vi "Autonomous Independent.vi"() -> ()   [LabVIEW 2016]
doc: "This VI is called when autonomous begins, and will automatically be terminated when autonomous ends. You can carry out timed or sensor driven robot movement independently without needing to return to the caller."
uses:
  <vilib>/Rock Robotics/WPI/Utilities/WPI_GetSetVariantRefNum.vi
  <vilib>/Rock Robotics/Network Tables/NT Read String.vi
  <vilib>/Rock Robotics/WPI/RobotDrive/WPI_RobotDriveArcadeDrive_Standard(NoSaturation).vi
  <vilib>/Rock Robotics/Network Tables/NT Write Numeric Array.vi
  <vilib>/Rock Robotics/WPI/Solenoid/WPI_SolenoidValue.ctl
  <vilib>/Rock Robotics/WPI/Solenoid/WPI_SolenoidSetEnum.vi
panel:
  in  "stop":bool
  in  "Left":dbl=0.5 step=0.1 format="%#_13g"
  in  "Right":dbl=0.45 step=0.1 format="%#_13g"
  # "Be sure to right-click and choose Data Operations>>Make Current Value default if you want to save the array values with the VI"
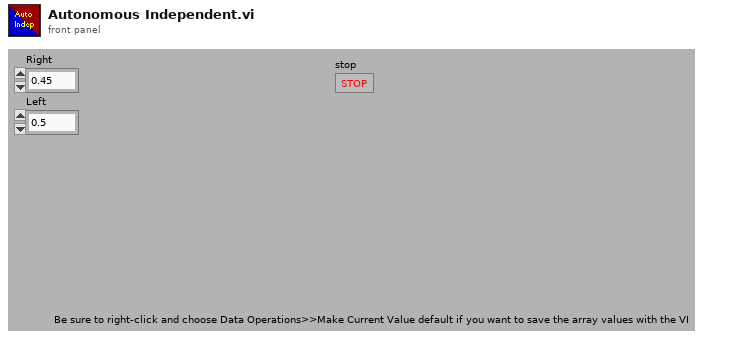
[diagram p1: front panel]
types:
  T1 = typedef "WPI_JoystickDevRef.ctl" = cluster{"Device":T2}
  T2 = typedef "WPI_JoystickDeviceEnum.ctl" = enum16{"USB 0", "USB 1", "USB 2", "USB 3", "USB 4", "USB 5"}
  T3 = typedef "WPI_SolenoidValue.ctl" = enum16{"Off", "On", "Forward", "Reverse"}
  T4 = typedef "WPI_SolenoidDevRef.ctl" = cluster{"DevStatus":errorcluster, "Pneumatics Control Module":u8, "Forward Solenoid Channel":T5, "Reverse Solenoid Channel":T5}
  T5 = typedef "WPI_SolenoidChannel.ctl" = enum8{"Solenoid 0", "Solenoid 1", "Solenoid 2", "Solenoid 3", "Solenoid 4", "Solenoid 5", "Solenoid 6", "Solenoid 7", "Invalid"}
  T6 = typedef "WPI_RobotDriveDevRef.ctl" = cluster{"DevStatus":errorcluster, "Motors[]":T7[], "Square Inputs":bool, "Max Output":dbl}
  T7 = typedef "WPI_MotorControlDeviceRef.ctl" = cluster{"DeviceStatus":errorcluster, "Type":T8, "PWM":cluster{"PWM Channel":T9, "DeadBand":T10}, "CAN":cluster{"Device Number":u8, "SetOutput VI Ref":variant, "GetOutput VI Ref":variant, "Enable VI Ref":variant, "Disable VI Ref":variant, "Data":variant}, "Invert":bool}
  T8 = typedef "WPI_MotorControlType.ctl" = enum16{"PWM", "CAN"}
  T9 = typedef "FPGA_DIOPWMChannel.ctl" = enum8{"PWM 0", "PWM 1", "PWM 2", "PWM 3", "PWM 4", "PWM 5", "PWM 6", "PWM 7", "PWM 8", "PWM 9", "PWM MXP 0", "PWM MXP 1", "PWM MXP 2", "PWM MXP 3", "PWM MXP 4", "PWM MXP 5", "PWM MXP 6", "PWM MXP 7", "PWM MXP 8", "PWM MXP 9", "Invalid"}
  T10 = typedef "WPI_PWMDeadband.ctl" = cluster{"Name":string, "maxPositivePwm":i32, "minPositivePwm":i32, "centerPwm":i32, "maxNegativePwm":i32, "minNegativePwm":i32, "angularRange":u16}
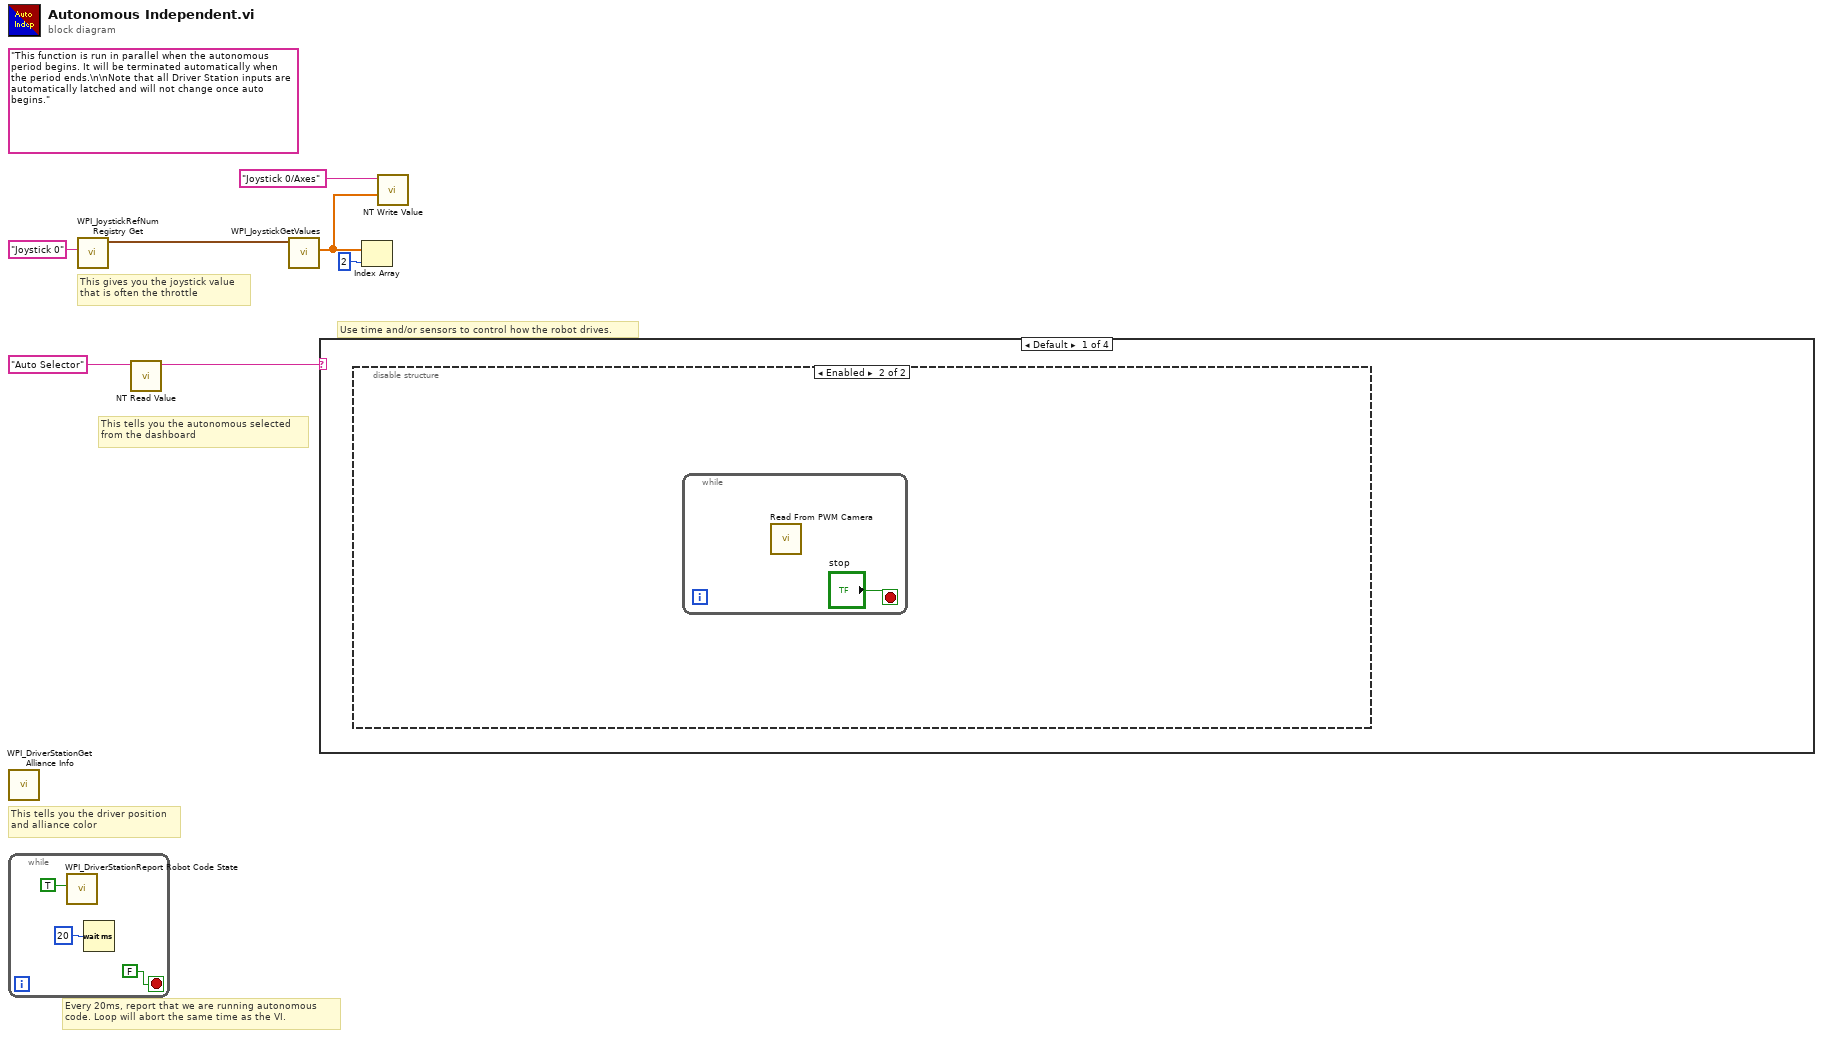
[diagram p0: block diagram]
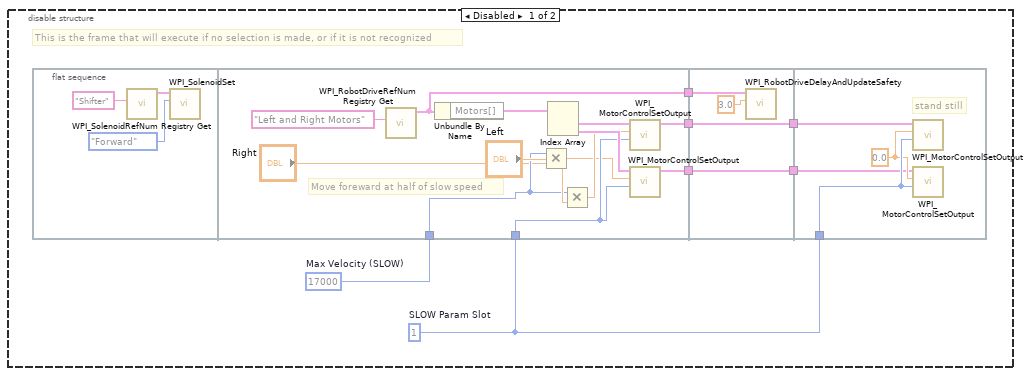
[diagram p2: hidden frame]
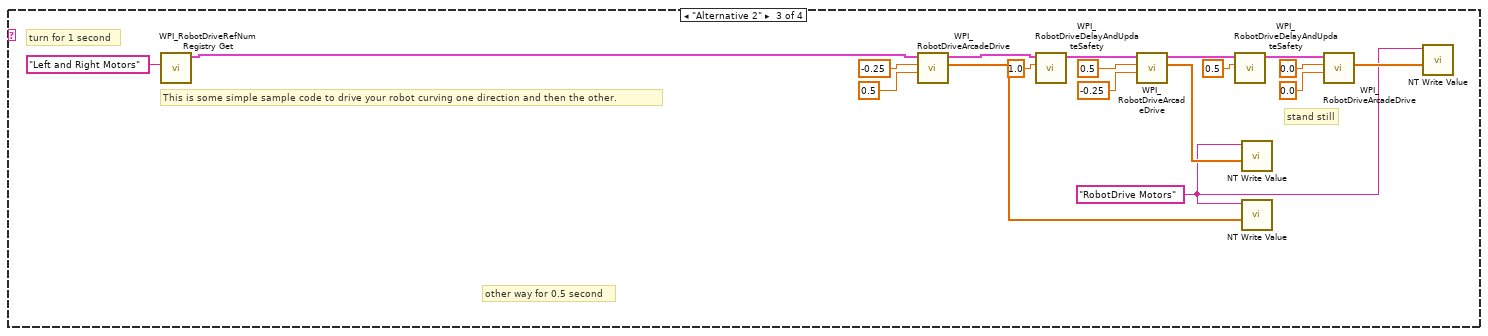
[diagram p4: hidden frame]
diagram:
  (unwired) "This function is run in parallel when the autonomous period begins. It will be terminated automatically when the period ends.\n\nNote that all Driver Station inputs are automatically latched and will not change once auto begins."
  # "This tells you the autonomous selected\nfrom the dashboard"
  # "Every 20ms, report that we are running autonomous\ncode. Loop will abort the same time as the VI."
  # "This gives you the joystick value\nthat is often the throttle"
  # "Use time and/or sensors to control how the robot drives."
  # "This tells you the driver position\nand alliance color"
  n1 = call <vilib>:"WPI_DriverStationGet Alliance Info.vi"() -> ()  [unwired: 12 out]
  n2 = while {
    stop <- FALSE stop-if-true
    n3 = call <vilib>:"WPI_DriverStationReport Robot Code State.vi"("Autonomous"=TRUE) -> ()  [unwired: 10 in, 1 out]
    n4 = Wait (ms)(milliseconds to wait=u32 20) -> ()  [unwired: 1 out]
  }
  n5 = call <vilib>:"WPI_JoystickRefNum Registry Get.vi"("refnum name"="Joystick 0") -> ("JoystickDevRef"=w6:T1)  [unwired: 1 in, 9 out]
  n6 = call-poly <vilib>:"NT Read Value.vi"("Name"="Auto Selector") -> ("String"=w3:string)  [unwired: 9 in, 1 out]
  n7 = call <vilib>:"WPI_JoystickGetValues.vi"("JoystickDevRef"=w6) -> ("Axes"=w2:dbl[])  [unwired: 6 in, 4 out]
  n8 = case shown="Default" w3 {
    frame Default {
      n9 = disable-structure shown="Enabled" {
        frame Disabled {
          w12 = 17000  # Max Velocity (SLOW)
          w11 = 1  # SLOW Param Slot
          # "This is the frame that will execute if no selection is made, or if it is not recognized"
          n10 = flat-sequence {
            tunnel: [w30] -> w17
            tunnel: w11 -> [w27]
            tunnel: w12 -> [w23]
            tunnel: [w25] -> w16
            tunnel: [w24] -> w15
            tunnel: w17 -> [w36]
            tunnel: w16 -> [w35]
            tunnel: [w35] -> w14
            tunnel: w15 -> [w34]
            tunnel: [w34] -> w13
            tunnel: w11 -> [w41]
            tunnel: w14 -> [w39]
            tunnel: w13 -> [w38]
            frame #0 {
              n11 = call <vilib>:"WPI_SolenoidRefNum Registry Get.vi"("refnum name"="Shifter") -> ("SolenoidDevRef"=w19:T4)  [unwired: 9 in, 1 out]
              n12 = call-poly <vilib>:"WPI_SolenoidSet.vi"("Value"=WPI_SolenoidValue."Forward", "SolenoidDevRef"=w19) -> ()  [unwired: 8 in, 2 out]
            }
            frame #1 {
              # "Move foreward at half of slow speed"
              n13 = call <vilib>:"WPI_RobotDriveRefNum Registry Get.vi"("refnum name"="Left and Right Motors") -> ("RobotDriveDevRef"=w30:T6)  [unwired: 1 in, 9 out]
              n14 = Unbundle By Name(w30) -> ("Motors[]"=w31:T7[])
              n15 = Multiply(x=w23, y="Right") -> (x*y=w22:dbl)
              n16 = Index Array(array=w31) -> (element #1=w29:T7, element #2=w32:T7)  [unwired: 2 in]
              n17 = Multiply(x=w23, y="Left") -> (x*y=w28:dbl)
              n18 = call <vilib>:"WPI_MotorControlSetOutput.vi"("options"=w27, "Output"=w28, "MotorControlDevRef"=w29) -> ("MotorControlDevRef"=w25:T7)  [unwired: 6 in, 2 out]
              n19 = call <vilib>:"WPI_MotorControlSetOutput.vi"("options"=w27, "Output"=w22, "MotorControlDevRef"=w32) -> ("MotorControlDevRef"=w24:T7)  [unwired: 6 in, 2 out]
            }
            frame #2 {
              n20 = call <vilib>:"WPI_RobotDriveDelayAndUpdateSafety.vi"("Delay (s)"=3.0, "RobotDriveDevRef"=w36) -> ()  [unwired: 8 in, 2 out]
            }
            frame #3 {
              w40 = 0.0 ("Output")
              # "stand still"
              n21 = call <vilib>:"WPI_MotorControlSetOutput.vi"("options"=w41, "Output"=w40, "MotorControlDevRef"=w39) -> ()  [unwired: 6 in, 3 out]
              n22 = call <vilib>:"WPI_MotorControlSetOutput.vi"("options"=w41, "Output"=w40, "MotorControlDevRef"=w38) -> ()  [unwired: 6 in, 3 out]
            }
          }
        }
        frame Enabled {
          n23 = while {
            stop <- "stop" stop-if-true
            n24 = call "Read From PWM Camera.vi"() -> ()  [unwired: 9 in, 3 out]
          }
        }
      }
    }
    frame "Alternative 1" {
      # "This sample code describes robot movements in an array. You can extend it to control other motors\non your robot. You can also use file I/O to move the data to a text file."
    }
    frame "Alternative 2" {
      w44 = "RobotDrive Motors" ("Name")
      # "This is some simple sample code to drive your robot curving one direction and then the other."
      # "stand still"
      # "other way for 0.5 second"
      # "turn for 1 second"
      n25 = call <vilib>:"WPI_RobotDriveRefNum Registry Get.vi"("refnum name"="Left and Right Motors") -> ("RobotDriveDevRef"=w60:T6)  [unwired: 1 in, 9 out]
      n26 = call-poly <vilib>:"WPI_RobotDriveArcadeDrive.vi"("Y axis value"=0.5 ("X axis value"), "X axis value"=-0.25, "RobotDriveDevRef"=w60) -> ("Motor Values"=w43:dbl[], "RobotDriveDevRef"=w53:T6)  [unwired: 1 in, 6 out]
      n27 = call <vilib>:"WPI_RobotDriveDelayAndUpdateSafety.vi"("Delay (s)"=1.0, "RobotDriveDevRef"=w53) -> ("RobotDriveDevRef 2"=w54:T6)  [unwired: 8 in, 1 out]
      n28 = call-poly <vilib>:"WPI_RobotDriveArcadeDrive.vi"("Y axis value"=-0.25 ("X axis value"), "X axis value"=0.5, "RobotDriveDevRef"=w54) -> ("Motor Values"=w45:dbl[], "RobotDriveDevRef"=w55:T6)  [unwired: 1 in, 6 out]
      n29 = call <vilib>:"WPI_RobotDriveDelayAndUpdateSafety.vi"("Delay (s)"=0.5, "RobotDriveDevRef"=w55) -> ("RobotDriveDevRef 2"=w56:T6)  [unwired: 8 in, 1 out]
      n30 = call-poly <vilib>:"NT Write Value.vi"("Numeric Array"=w45, "Name"=w44) -> ()  [unwired: 9 in, 1 out]
      n31 = call-poly <vilib>:"NT Write Value.vi"("Numeric Array"=w43, "Name"=w44) -> ()  [unwired: 9 in, 1 out]
      n32 = call-poly <vilib>:"WPI_RobotDriveArcadeDrive.vi"("Y axis value"=0.0 ("X axis value"), "X axis value"=0.0, "RobotDriveDevRef"=w56) -> ("Motor Values"=w46:dbl[])  [unwired: 1 in, 7 out]
      n33 = call-poly <vilib>:"NT Write Value.vi"("Numeric Array"=w46, "Name"=w44) -> ()  [unwired: 9 in, 1 out]
    }
    frame "Your Turn" {
    }
  }
  n34 = Index Array(array=w2, index=2) -> ()  [unwired: 1 out]
  n35 = call-poly <vilib>:"NT Write Value.vi"("Numeric Array"=w2, "Name"="Joystick 0/Axes") -> ()  [unwired: 9 in, 1 out]
